vi "Contains.vi"(8 "error in (no error)":errorcluster, 10 "Key":string, 11 "StringMap in":refnum<class "StringMap.lvclass">) -> (0 "error out":errorcluster, 1 "Key Exists?":bool, 3 "StringMap out":refnum<class "StringMap.lvclass">)   [LabVIEW 2013, in "LapDog.Collections.v1.Maps.lvlib" / "StringMap.lvclass"]
doc: "Returns a boolean True if the key exists in the map."
uses:
  StringMap.lvclass
  StringMap.lvclass/StringMap.ctl
  ObjectMap/ObjectMap.lvclass
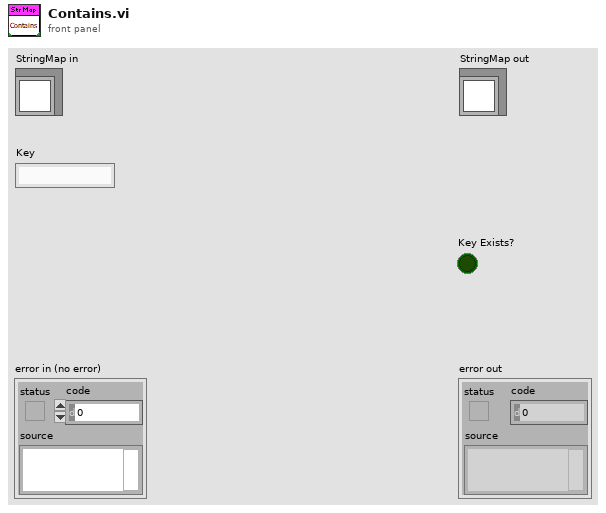
[diagram p1: front panel]
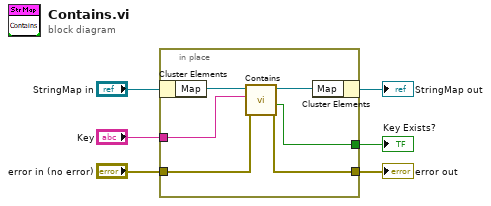
[diagram p0: block diagram]
diagram:
  n1 = in-place {
    in-place-border: "Key" -> [w10]
    in-place-border: "error in (no error)" -> [w9]
    in-place-border: [w8] -> w3
    in-place-border: [w7] -> w2
    n2 = in-place-cluster #1("StringMap in") -> ("Map"=w12:refnum<class "ObjectMap.lvclass">)
    n3 = call-dynamic "Contains.vi"("error in (no error)"=w9, "Key"=w10, "Map in"=w12) -> ("error out"=w8:errorcluster, "Key Exists?"=w7:bool, "Map out"=w11:refnum<class "ObjectMap.lvclass">)  [unwired: 6 in]
    n4 = in-place-cluster #1("Map"=w11) -> (→"StringMap out":refnum<class "StringMap.lvclass">)
  }
  "error out" <- w3
  "Key Exists?" <- w2
